vi "Binary Decoder.vi"(1 "Number":u64) -> (0 "Bits":bool[](array[boolean]))   [LabVIEW 2016]
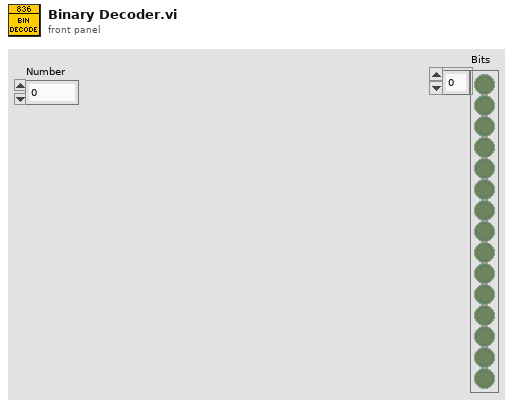
[diagram p1: front panel]
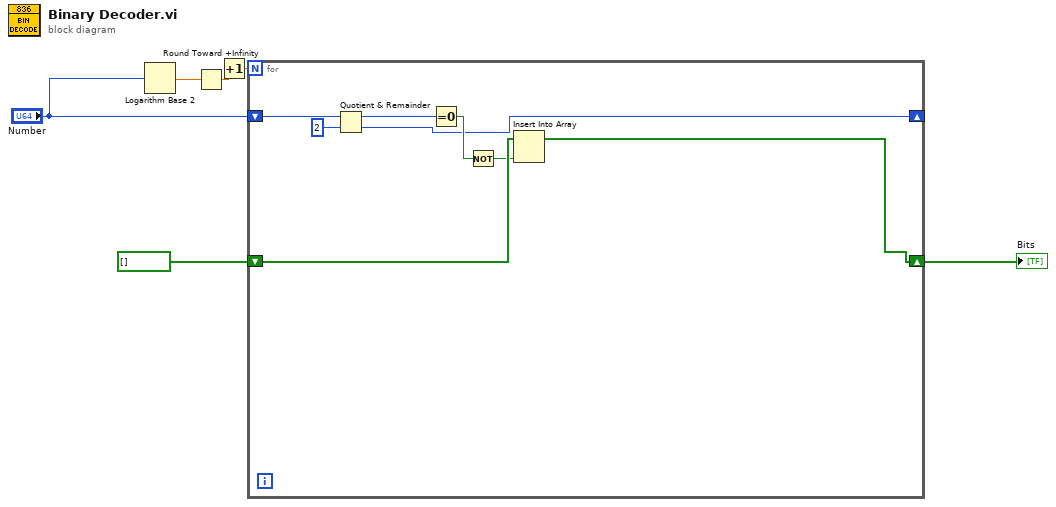
[diagram p0: block diagram]
diagram:
  n1 = Logarithm Base 2(1:"Number") -> (0:w6:dbl)
  n2 = Round Toward +Infinity(x=w6) -> (ceil(x): smallest int >= x=w5:dbl)
  n3 = Increment(x=w5) -> (x+1=w1:dbl)
  n4 = for {
    N: w1 -> [_]
    shift-right: [w8] -> _
    shift-left: "Number" -> [w14]
    shift-right: [w9] -> w2
    shift-left: bool[] [] ("Bits") -> [w11]
    n5 = Quotient & Remainder(x=w14, y=u64 2) -> (x-y*floor(x/y)=w12:u64, floor(x/y)=w8:u64)
    n6 = Equal To 0?(x=w12) -> (x = 0?=w10:bool)
    n7 = Not(x=w10) -> (.not. x?=w7:bool)
    n8 = Insert Into Array(array=w11, new element=w7) -> (w9:bool[])  [unwired: 1 in]
  }
  "Bits" <- w2
